vi "Attente_Tempo_Handler.vi"(8 "Error In":errorcluster caption="Entrée d'erreur", 11 "Donnees_Globales_IN":T1) -> (0 "Error Out":errorcluster caption="Sortie d'erreur", 3 "Donnees_Globale_Out":T1)   [LabVIEW 2019]
uses:
  Asc_State_Inputs.ctl
  Etat_Asc.ctl
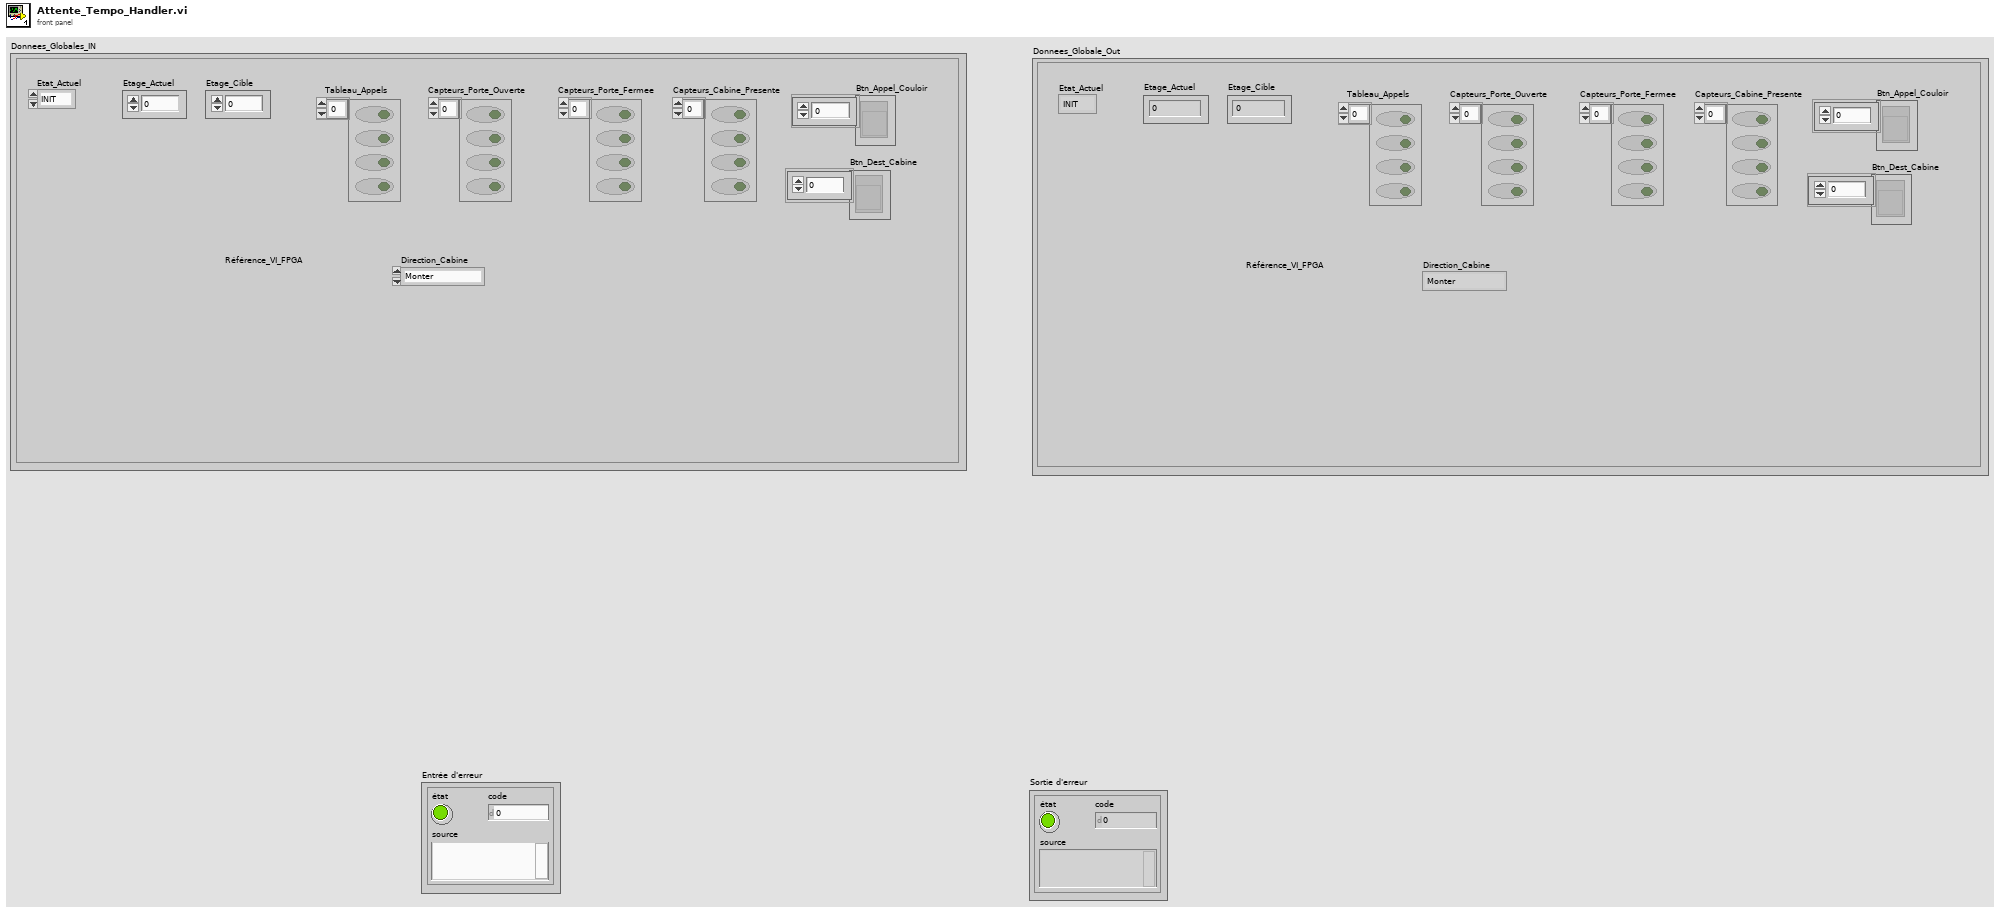
[diagram p1: front panel]
types:
  T1 = typedef "Asc_State_Inputs.ctl" = cluster{"Etage_Actuel":i32, "Etat_Actuel":T2, "Etage_Cible":i32, "Tableau_Appels":bool[], "Capteurs_Porte_Ouverte":bool[], "Capteurs_Porte_Fermee":bool[], "Capteurs_Cabine_Presente":bool[], "Btn_Appel_Couloir":refnum<vi>[], "Btn_Dest_Cabine":refnum<vi>[], "Référence_VI_FPGA":refnum<k20>, "Direction_Cabine":enum16{"Monter", "Descendre", "Arreter"}}
  T2 = typedef "Etat_Asc.ctl" = enum16{"INIT", "REPOS", "DEPLACEMENT", "OUVERTURE_PORTE", "ATTENTE_TEMPO", "FERMETURE_PORTE", "ARRET_URGENCE"}
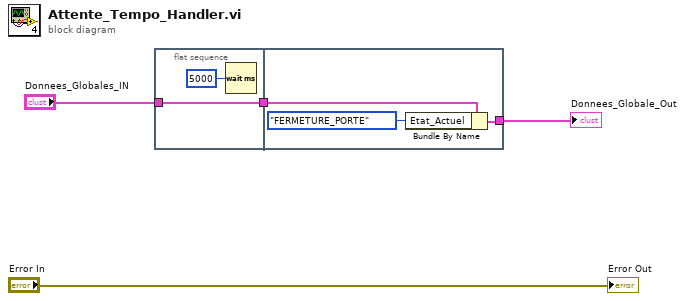
[diagram p0: block diagram]
diagram:
  n1 = flat-sequence {
    tunnel: [w5] -> w3
    tunnel: "Donnees_Globales_IN" -> [w5]
    tunnel: w3 -> [w8]
    tunnel: [w7] -> w1
    frame #0 {
      n2 = Wait (ms)(milliseconds to wait=u32 5000 ("attente (ms)")) -> ()  [unwired: 1 out]
    }
    frame #1 {
      n3 = Bundle By Name(cluster=w8, "Etat_Actuel"=Etat_Asc."FERMETURE_PORTE") -> (w7:T1)
    }
  }
  "Donnees_Globale_Out" <- w1
  "Error Out" <- "Error In"
